vi "ARydh_set_frequency -- V1.vi"(4 "Oscillator (0)":u16, 8 "Error In":errorcluster, 9 "timeconstant (s)":dbl=0.006, 10 "Freq in (Hz)":dbl=40000.0 format="%#_13g", 11 "MCL object":T1) -> (0 "Error Out":errorcluster, 1 "z out (V)":cdb, 2 "Freq out (Hz)":dbl=40000.0 format="%#_13g", 3 "MCL object OUT":T1)   [LabVIEW 2020]
uses:
  nanocal/Nanocalorimetry/data/MCL.lvlibp/SynkTek FPGA/FPGA_SharedResources/FPGASharedResources_FreqCtrl_FreqGenTypedef.ctl
  nanocal/Nanocalorimetry/data/MCL.lvlibp/SynkTek Host/LIControl/LIControl_LockinTimeConstant_typedef.ctl
  nanocal/Nanocalorimetry/data/MCL.lvlibp/SynkTek Host/LIControl/LIControl_FreqCtrl_typedef.ctl
  nanocal/Nanocalorimetry/data/MCL.lvlibp/SynkTek FPGA/FPGA_SharedResources/FPGASharedResources_PhaseShiftCtrl_Typedef.ctl
  nanocal/Nanocalorimetry/data/MCL.lvlibp/MCL library/MCL_DataRef.ctl
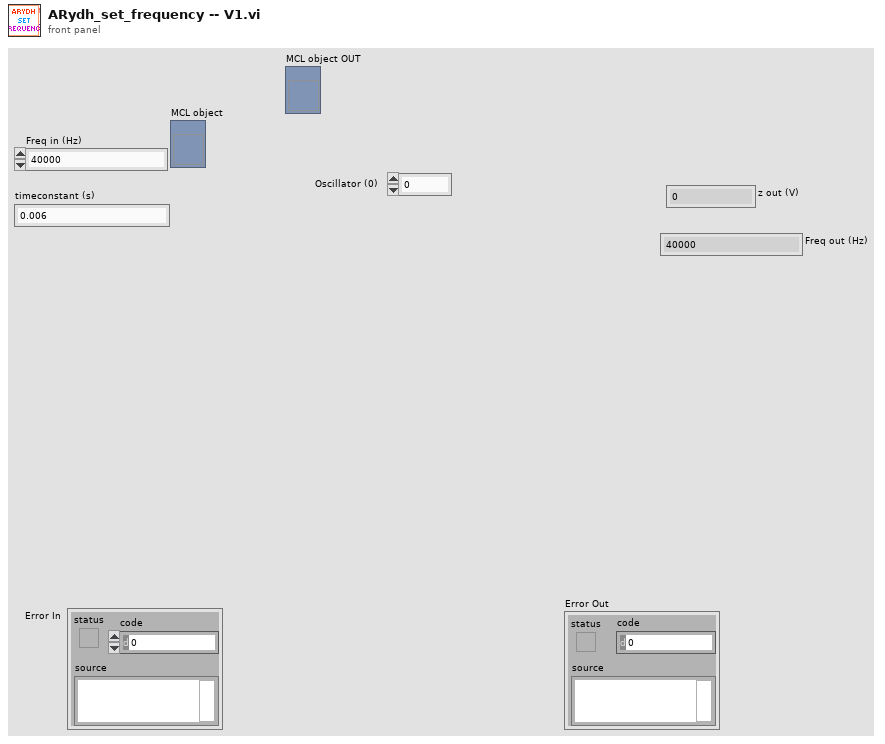
[diagram p1: front panel]
types:
  T1 = typedef "MCL.lvlibp/MCL_DataRef.ctl" = refnum<vi>
  T2 = typedef "MCL.lvlibp/FPGA_SharedResources.lvlib/FPGASharedResources_PhaseShiftCtrl_Typedef.ctl" = enum8{"Phase 1", "Phase 2", "Phase 3", "Phase 4", "Phase 5", "Phase 6", "Phase 7", "Disabled"}
  T3 = typedef "MCL.lvlibp/FPGA_SharedResources.lvlib/FPGASharedResources_FreqCtrl_FreqGenTypedef.ctl" = enum8{"Frequency 1", "Frequency 2", "Frequency 3", "Frequency 4", "Frequency 5", "Frequency 6: PLL 1", "Frequency 7: PLL 2", "Frequency 8"}
  T4 = typedef "MCL.lvlibp/LIControl.lvlib/LIControl_FreqCtrl_typedef.ctl" = cluster{"Frequency (Hz)":dbl, "Ramp changes":bool, "Ramp time const. (s)":T5}
  T5 = typedef "MCL.lvlibp/LIControl.lvlib/LIControl_LockinTimeConstant_typedef.ctl" = dbl
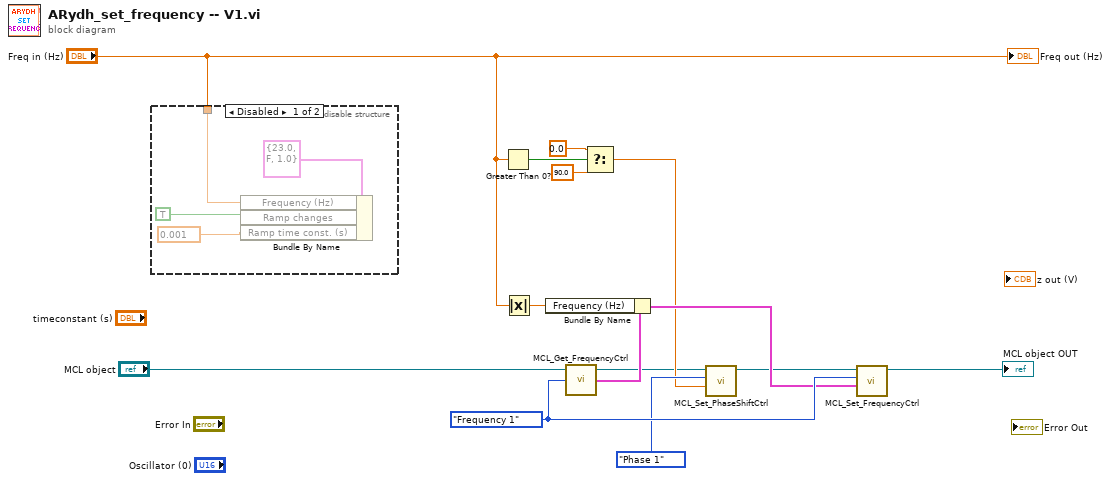
[diagram p0: block diagram]
diagram:
  w12 = FPGASharedResources_FreqCtrl_FreqGenTypedef."Frequency 1" ("Frequency generator")
  n1 = disable-structure shown="Disabled" {
    disable-tunnel: "Freq in (Hz)" -> [w15 _]
    frame Disabled {
      w16 = T5 0.001 items=["100 s"=100.0, "50 s"=50.0, "20 s"=20.0, "10 s"=10.0, "5 s"=5.0, "3 s"=3.0, "2 s"=2.0, "1 s"=1.0, "0.5 s"=0.5, "0.3 s"=0.3, "0.2 s"=0.2, "0.1 s"=0.1, "50 ms"=0.05, "20 ms"=0.02, "10 ms"=0.01, "5 ms"=0.005, "2 ms"=0.002, "1 ms"=0.001] ("Ramp time const. (s)")
      n2 = Bundle By Name(cluster=T4 {"Frequency (Hz)"=23.0, "Ramp changes"=FALSE, "Ramp time const. (s)"=1.0} ("FrequencyCtrl"), "Frequency (Hz)"=w15, "Ramp changes"=TRUE, "Ramp time const. (s)"=w16) -> ()  [unwired: 1 out]
    }
    frame Enabled {
    }
  }
  n3 = Greater Than 0?(x="Freq in (Hz)") -> (x > 0?=w6:bool)
  n4 = Absolute Value(x="Freq in (Hz)") -> (abs(x)=w8:dbl)
  n5 = call "MCL_Get_FrequencyCtrl.vi"("Frequency generator"=w12, "MCL object"="MCL object") -> ("FrequencyCtrl"=w11:T4, "MCL object"=w2:T1)  [unwired: 1 in, 1 out]
  n6 = Bundle By Name(cluster=w11, "Frequency (Hz)"=w8) -> (w10:T4)
  n7 = Select(t=0.0, s=w6, f=90.0) -> (s? t:f=w3:dbl)
  n8 = call "MCL_Set_PhaseShiftCtrl.vi"("Phase shift (deg)"=w3, "Phase shift"=FPGASharedResources_PhaseShiftCtrl_Typedef."Phase 1", "MCL object"=w2) -> ("MCL object"=w1:T1)  [unwired: 3 in, 1 out]
  n9 = call "MCL_Set_FrequencyCtrl.vi"("FrequencyCtrl"=w10, "Frequency generator"=w12, "MCL object"=w1) -> ("MCL object"=→"MCL object OUT":T1)  [unwired: 3 in, 1 out]
  "Freq out (Hz)" <- "Freq in (Hz)"
